vi "Parse Body.vi"(8 "error in":errorcluster, 10 "HTTP Status in":T2, 11 "Header-Body Data in":T1) -> (0 "error out":errorcluster, 2 "HTTP Status out":T2, 3 "Header-Body Data out":T1)   [LabVIEW 2020, in "InfluxDB v2 Client.lvlib"]
doc: "Parses the body into the components:\n1) Status\n2) Desciption"
uses:
  InfluxDB v2 Client.lvlib
  HTTP Status.ctl
  Header-Body Data.ctl
  <vilib>/LVH/i3 JSON/JSON Parsing/Get Object Parameter Files/Get Object Parameter - String.vi
  <vilib>/LVH/i3 JSON/i3-json.lvlib
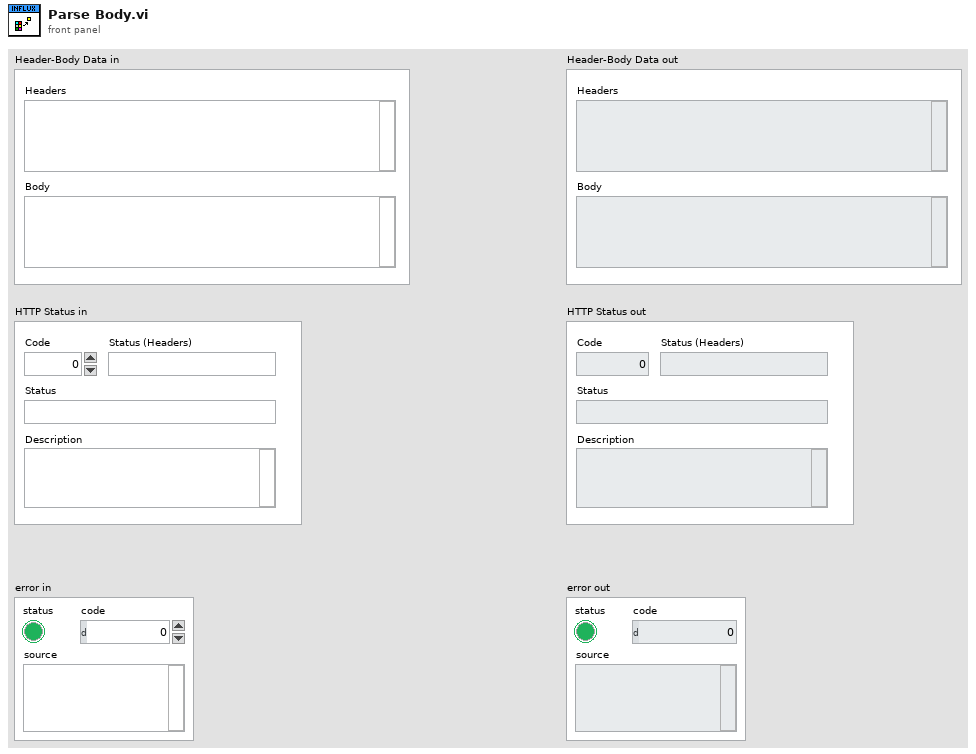
[diagram p1: front panel]
types:
  T1 = typedef "InfluxDB v2 Client.lvlib/Header-Body Data.ctl" = cluster{"Headers":string, "Body":string}
  T2 = typedef "InfluxDB v2 Client.lvlib/HTTP Status.ctl" = cluster{"Code":i32, "Status":string, "Description":string, "Status (Headers)":string}
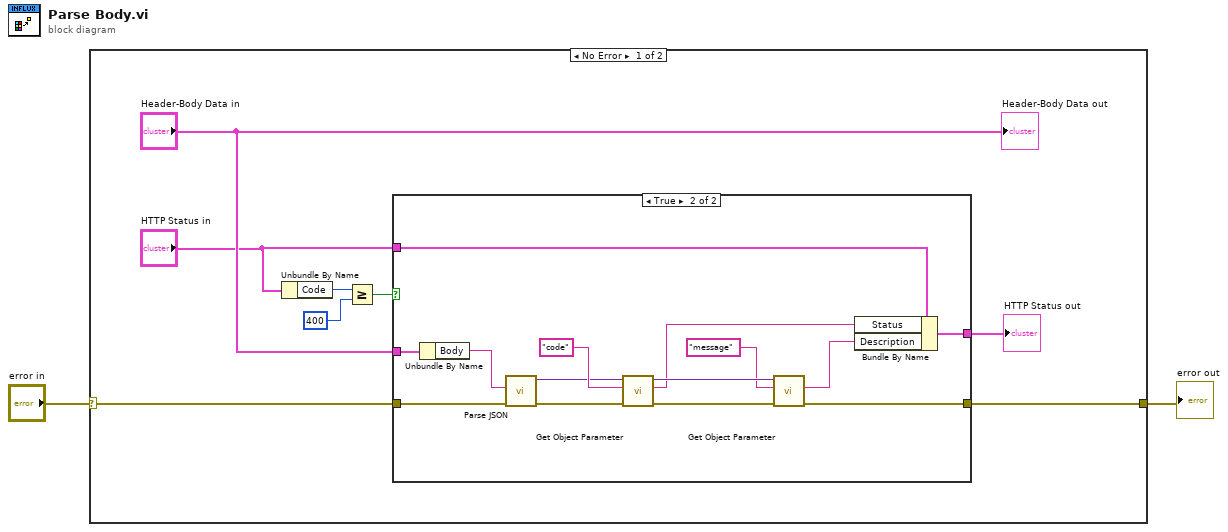
[diagram p0: block diagram]
diagram:
  n1 = case shown="No Error" "error in" {
    selector: "error in" -> [w9 w27]
    tunnel: [w10 w27] -> w1
    frame No Error {
      n2 = Unbundle By Name("HTTP Status in") -> ("Code"=w6:i32)
      n3 = Greater Or Equal?(x=w6, y=400) -> (x >= y?=w4:bool)
      n4 = case shown="True" w4 {
        tunnel: [w11 w18] -> w10
        tunnel: w9 -> [w11 w17]
        tunnel: "Header-Body Data in" -> [_ w16]
        tunnel: "HTTP Status in" -> [w12 w14]
        tunnel: [w12 w13] -> w3
        frame False {
        }
        frame True {
          n5 = Unbundle By Name(w16) -> ("Body"=w26:string)
          n6 = call <vilib>:"Parse JSON.vi"("error in (no error)"=w17, "JSON String"=w26) -> ("error out"=w24:errorcluster, "JSON Tree"=w23:variant)  [unwired: 6 in, 2 out]
          n7 = call-poly <vilib>:"Get Object Parameter.vi"("error in (no error)"=w24, "Parameter Name"="code", "JSON Tree In (JSON Object)"=w23) -> ("error out"=w22:errorcluster, "String Value"=w19:string, "JSON Tree Out Passthrough"=w21:variant)  [unwired: 5 in, 1 out]
          n8 = call-poly <vilib>:"Get Object Parameter.vi"("error in (no error)"=w22, "Parameter Name"="message", "JSON Tree In (JSON Object)"=w21) -> ("error out"=w18:errorcluster, "String Value"=w15:string)  [unwired: 5 in, 2 out]
          n9 = Bundle By Name(cluster=w14, "Status"=w19, "Description"=w15) -> (w13:T2)
        }
      }
      "HTTP Status out" <- w3
      "Header-Body Data out" <- "Header-Body Data in"
    }
    frame Error {
    }
  }
  "error out" <- w1
